vi "FramesPerSecondTOMilliseconds.vi"(11 "Thermometer\nFps":dbl) -> (2 "x*y":dbl)   [LabVIEW 2016]
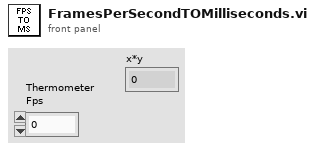
[diagram p1: front panel]
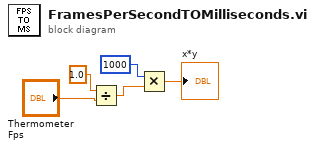
[diagram p0: block diagram]
diagram:
  n1 = Divide(x=1.0, y="Thermometer\nFps") -> (x/y=w4:dbl)
  n2 = Multiply(x=1000, y=w4) -> (x*y=→"x*y":dbl)
